vi "Coordinate_transforms.vi"(1 "Traverse Name":string="EnFlo Tunnel", 2 "Input":dbl[](array[numeric])=[0.0, 0.0, 0.0] format="%.2f", 3 "Mode":enum16{"XYZ to Channel", "Channel to XYZ"}(ring)) -> (0 "Output":dbl[](array[numeric]) format="%.2f")   [LabVIEW 2010]
uses:
  DriveConfigGlobal.vi
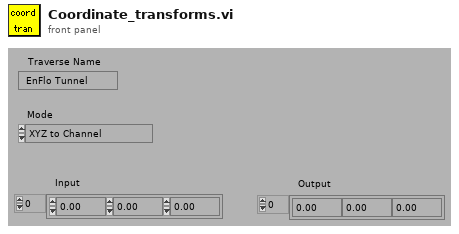
[diagram p1: front panel]
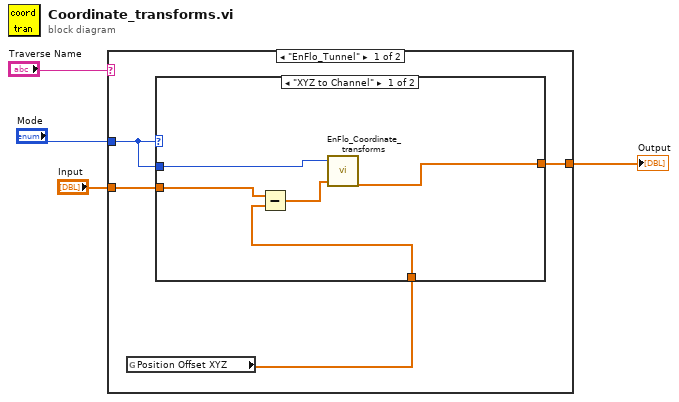
[diagram p0: block diagram]
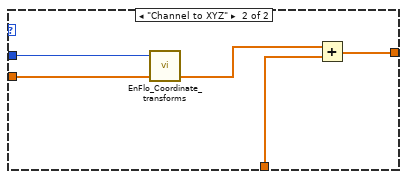
[diagram p2: hidden frame]
diagram:
  n1 = case shown="\"EnFlo_Tunnel\"" "Traverse Name" {
    tunnel: "Input" -> [w8 w19]
    tunnel: [w6 w19] -> w3
    tunnel: "Mode" -> [w5 _]
    frame "EnFlo_Tunnel" {
      n2 = global read "DriveConfigGlobal.vi" "Position Offset XYZ"() -> (w7:dbl[])
      n3 = case shown="\"XYZ to Channel\"" w5 {
        tunnel: w8 -> [w11 w18]
        tunnel: w7 -> [w12 w16]
        tunnel: [w10 w15] -> w6
        tunnel: w5 -> [w9 w14]
        frame "XYZ to Channel" {
          n4 = Subtract(x=w11, y=w12) -> (x-y=w13:dbl[])
          n5 = call "EnFlo_Coordinate_transforms.vi"("Input"=w13, "Mode"=w9) -> ("Output"=w10:dbl[])  [unwired: 3 out]
        }
        frame "Channel to XYZ" {
          n6 = call "EnFlo_Coordinate_transforms.vi"("Input"=w18, "Mode"=w14) -> ("Output"=w17:dbl[])  [unwired: 3 out]
          n7 = Add(x=w17, y=w16) -> (x+y=w15:dbl[])
        }
      }
    }
    frame "D_Tunnel", Default {
    }
  }
  "Output" <- w3
